vi "MakeHistogram.vi"(0 "Signal":dynamicdata(graph), 5 "Number of Bins":i32=10, 7 "Maximum Value":dbl=1.5e-07, 9 "Minimum Value":dbl, 11 "error in (no error)":errorcluster) -> (4 "Histogram":dynamicdata(graph), 15 "error out":errorcluster)   [LabVIEW 2013, in "GP22_TDC_Arduinoed.lvlib"]
doc: "Computes a histogram for <B>Signal</B>.\n--------------------\n\nThis Express VI is configured as follows:\n\nNumber of Bins: 10\nMinimum Value: 0\nMaximum Value: 1.5E-7\nAmplitude Representation: Sample Count"
uses:
  GP22_TDC_Arduinoed.lvlib
panel:
  out "Signals In":dynamicdata(graph)
  in  "Enable":bool=TRUE
  in  "Reset":bool=TRUE
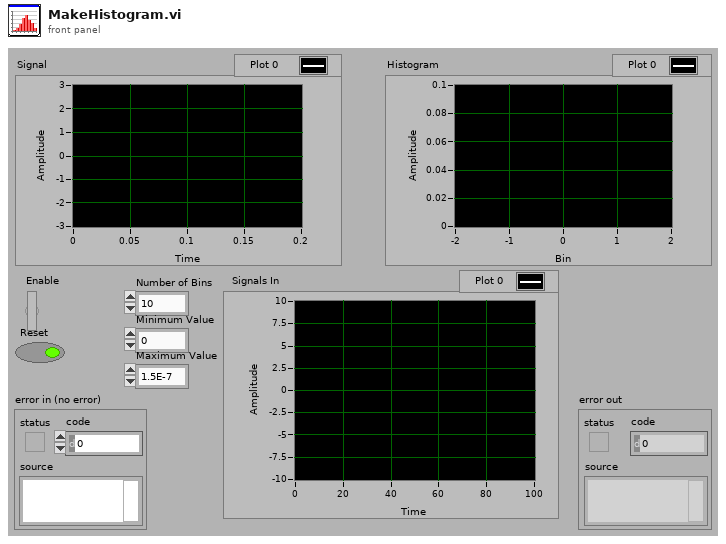
[diagram p1: front panel]
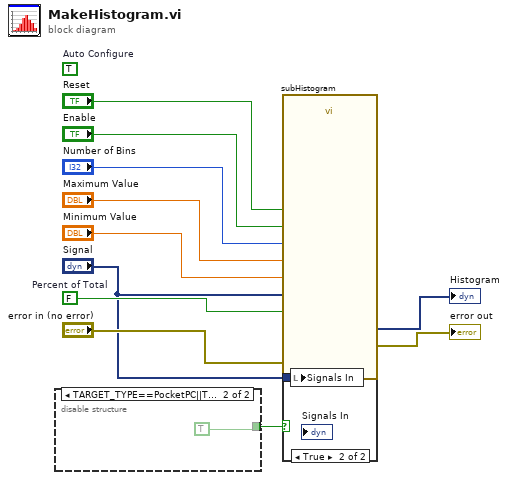
[diagram p0: block diagram]
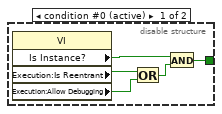
[diagram p2: hidden frame]
diagram:
  w6 = FALSE  # Percent of Total
  (unwired) TRUE  # Auto Configure
  n1 = disable-structure shown="TARGET_TYPE==PocketPC||TARGET_TYPE==PalmOS||TARGET_TYPE==Embedded" {
    disable-tunnel: [w16 TRUE] -> w2
    frame condition #0 (active) {
      n2 = property class="VI"() -> ("Is Instance?"=w15:bool, "Execution:Is Reentrant"=w13:bool, "Execution:Allow Debugging"=w12:bool)  [unwired: 2 in, 2 out]
      n3 = Or(x=w13, y=w12) -> (x .or. y?=w14:bool)
      n4 = And(x=w15, y=w14) -> (x .and. y?=w16:bool)
    }
    frame condition #1 {
    }
  }
  n5 = call <vilib>:"subHistogram.vi"("Enable"="Enable", "Percent of Total"=w6, "Reset"="Reset", "Number of Bins"="Number of Bins", "error in (no error)"="error in (no error)", "Maximum Value"="Maximum Value", "Minimum Value"="Minimum Value", "Input"="Signal") -> ("error out"=→"error out":errorcluster, "Histogram"=→"Histogram":dynamicdata)  [unwired: 2 in]
  n6 = case shown="True" w2 {
    tunnel: "Signal" -> [_ w18]
    frame False {
    }
    frame True {
      n7 = local write "Signals In"(w18) -> ()
    }
  }
